vi "波形生成与数据存储.vi"(6 "文件保存控制位":bool, 9 "数据输入":i32[][](array[numeric]), 10 "上一时刻时间输入":timestamp, 11 "文件存储地址":path) -> (1 "缓存区输出":i32[][](array[numeric]), 2 "时间输出":timestamp, 3 "输出波形":waveform(i32)[](graph))   [LabVIEW 2020]
uses:
  <vilib>/express/express analysis/Spectral/Block/exnSpectralBlock spectral measurements RMS poly.vi
  <vilib>/express/express analysis/Spectral/Block/exnSpectralBlock spectral measurements RMS WFM.vi
  <vilib>/express/express analysis/Spectral/XNode/ExpressSpectralMeasurementsBlockNode.xnode
panel:
  out "通道0频率分析示意":cluster{"f0":dbl, "df":dbl, "magnitude":dbl[]}(graph)
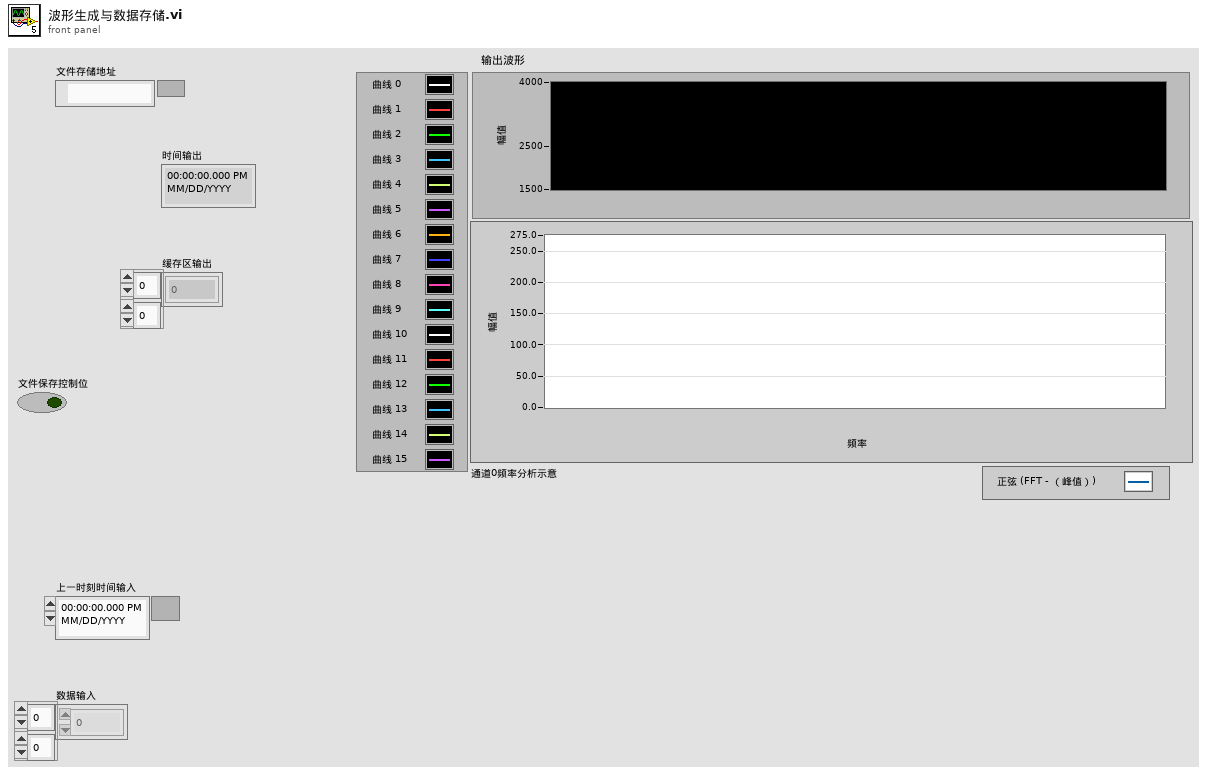
[diagram p1: front panel]
types:
  T1 = cluster{"averaging mode":u16, "weighting mode":u16, "number of averages":u32}
  T2 = cluster{"dB On (F)":bool, "unwrap phase (F)":bool, "convert to degree (F)":bool}
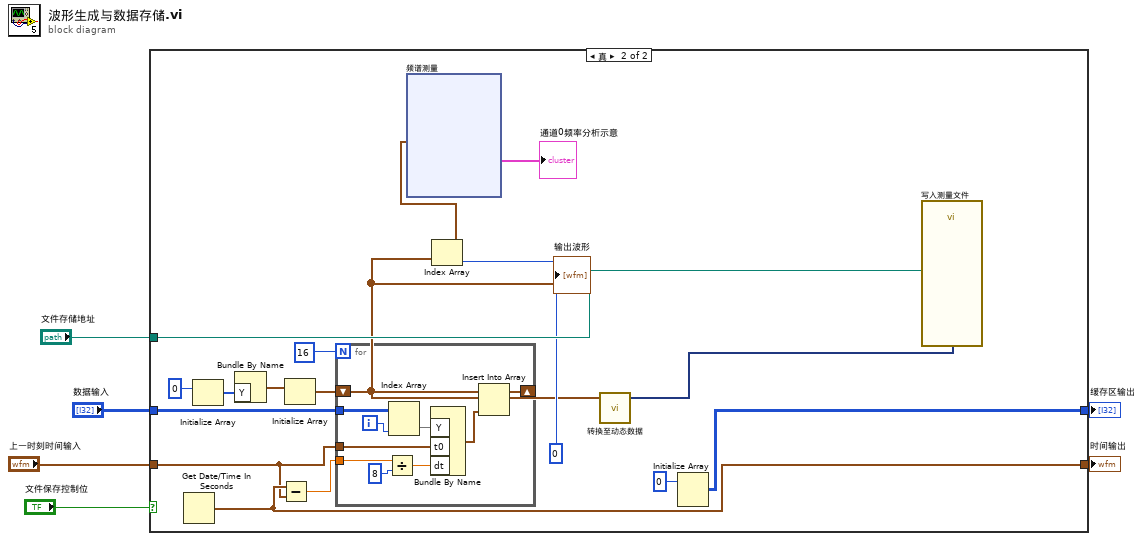
[diagram p0: block diagram]
diagram:
  n1 = case shown="真" "文件保存控制位" {
    tunnel: "数据输入" -> [w8 w16]
    tunnel: [w8 w24] -> w3
    tunnel: [w7 w15] -> w4
    tunnel: "上一时刻时间输入" -> [w7 w14]
    tunnel: "文件存储地址" -> [_ w13]
    frame False {
    }
    frame True {
      n2 = Get Date/Time In Seconds() -> (seconds since 1Jan1904=w15:timestamp)
      n3 = Initialize Array(0) -> (w19:i32[])  [unwired: 1 in]
      n4 = Bundle By Name ("创建波形")("Y"=w19) -> (w21:waveform(i32))  [unwired: 1 in]
      n5 = Subtract(x=w15, y=w14) -> (x-y=w18:dbl)
      n6 = Initialize Array(w21) -> (w22:waveform(i32)[])  [unwired: 1 in]
      n7 = for {
        N: 16 -> [_]
        shift-right: [w43] -> w11
        shift-left: w22 -> [w42]
        tunnel: w18 -> [w41]
        tunnel: w16 -> [w38]
        tunnel: w14 -> [w36]
        i -> [w45]
        n8 = Divide(x=w41, y=8) -> (x/y=w40:dbl)
        n9 = Index Array(array=w38, index (col)=w45) -> (element=w37:i32[])  [unwired: 1 in]
        n10 = Bundle By Name ("创建波形")("Y"=w37, "t0"=w36, "dt"=w40) -> (w44:waveform(i32))  [unwired: 1 in]
        n11 = Insert Into Array(array=w42, new element=w44) -> (w43:waveform(i32)[])  [unwired: 1 in]
      }
      "输出波形" <- w11
      n12 = Index Array(array=w11, index=0) -> (element=w9:waveform(i32))
      n13 = xnode "频谱测量"("信号"=w9) -> ("FFT - （均方根）"=→"通道0频率分析示意":cluster{"f0":dbl, "df":dbl, "magnitude":dbl[]})  [unwired: 1 in, 2 out]
      n14 = call "转换至动态数据"("Array of Waveforms"=w11) -> ("Dynamic Data Type"=w17:dynamicdata)  [unwired: 3 in]
      n15 = Initialize Array(0) -> (w24:i32[][])  [unwired: 2 in]
      n16 = call "写入测量文件"("Signals"=w17, "Filename"=w13) -> ()  [unwired: 15 in, 3 out]
    }
  }
  "时间输出" <- w4
  "缓存区输出" <- w3
